vi "LogCycleHistory.vi"(8 "error in (no error)":errorcluster, 11 "Cycle History String Data In":string[](array[string])) -> (0 "error out":errorcluster)   [LabVIEW 2016]
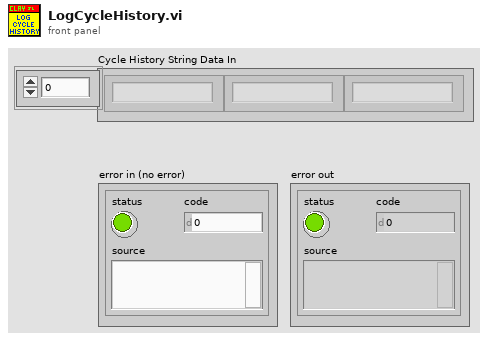
[diagram p1: front panel]
types:
  T1 = enum16{"open", "replace", "create", "open or create", "replace or create", "replace or create with confirmation"}
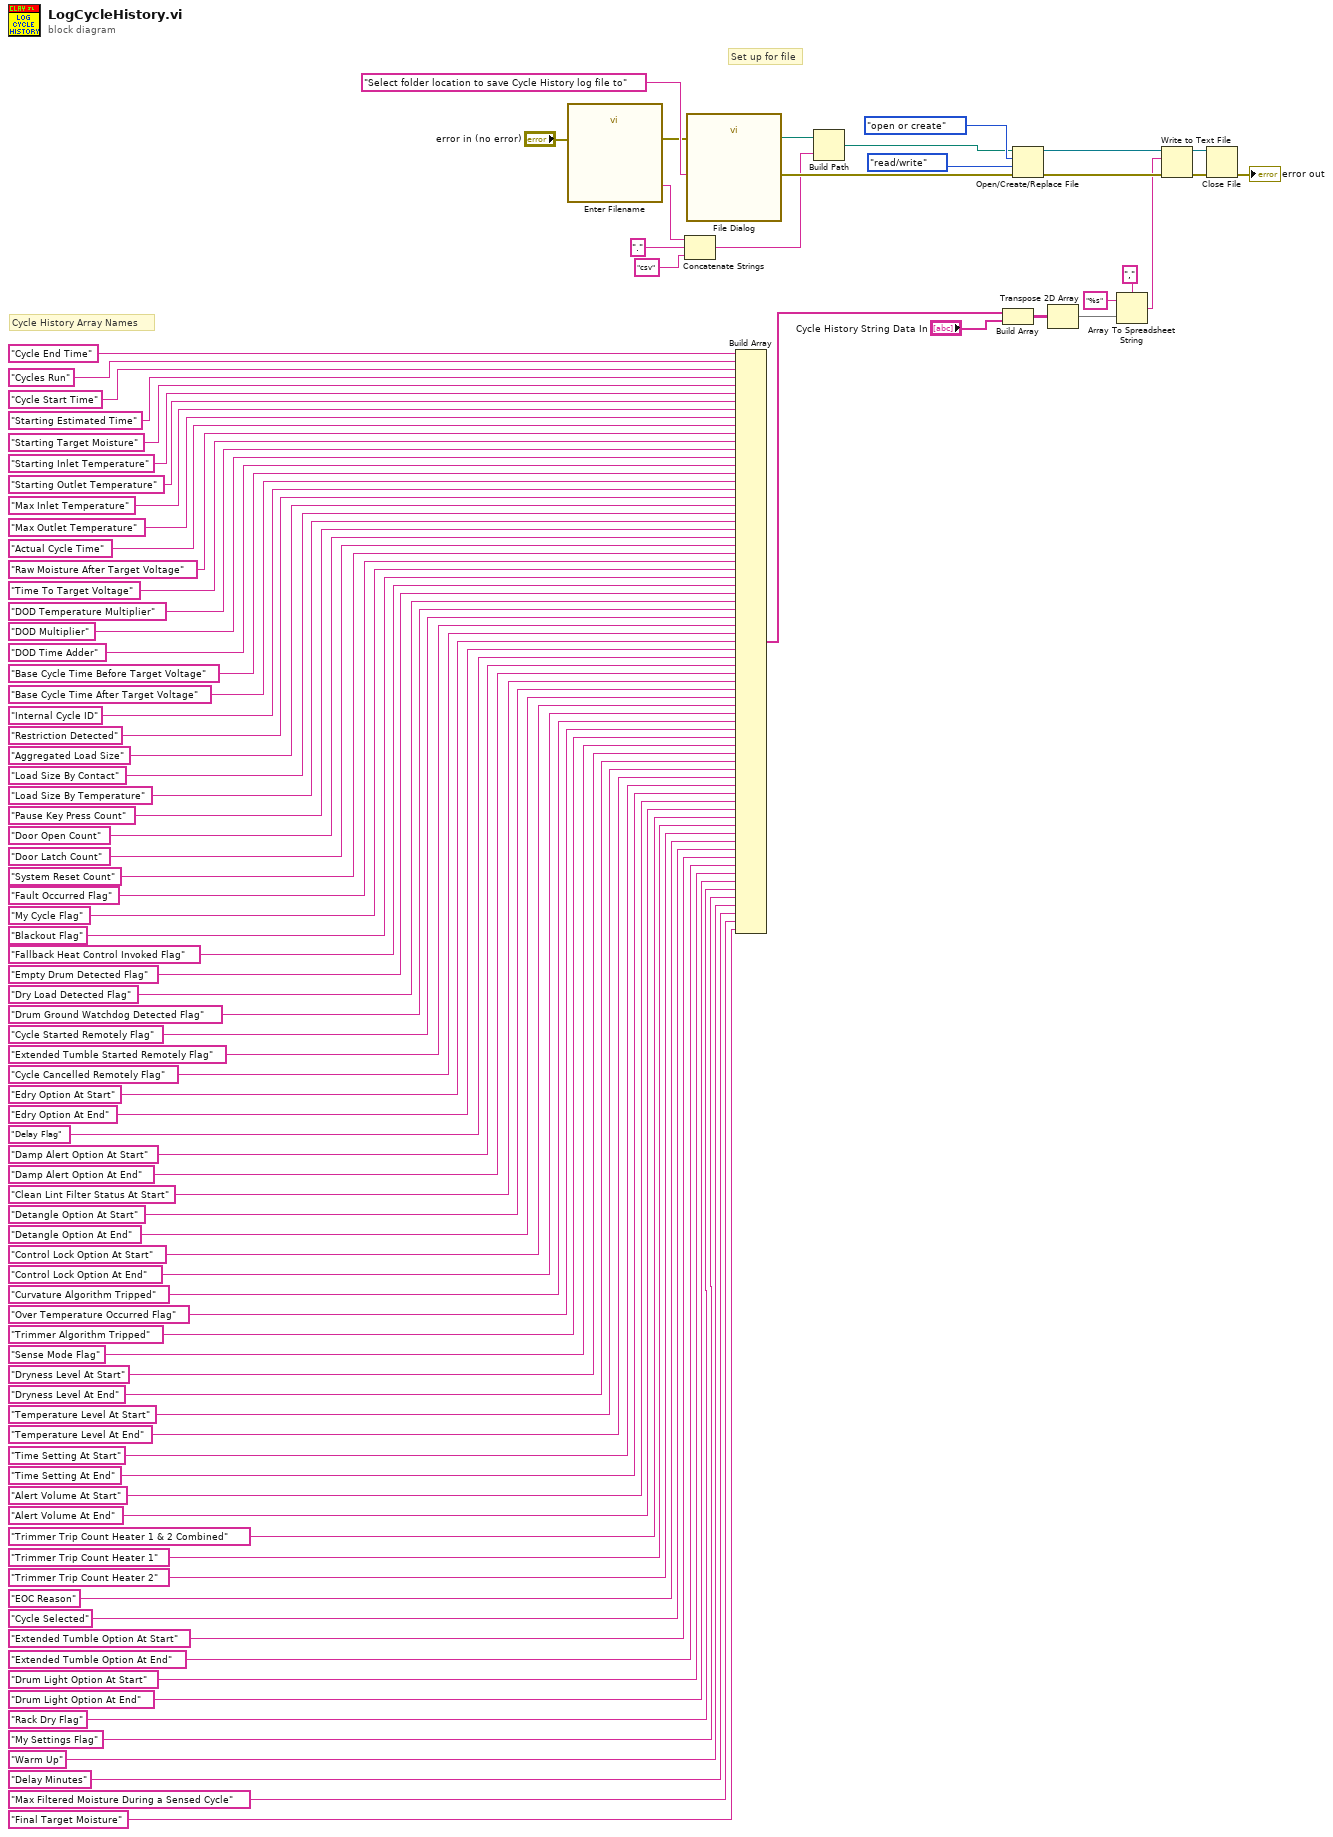
[diagram p0: block diagram]
diagram:
  # "Cycle History Array Names"
  # "Set up for file"
  n1 = call "Enter Filename"("error in (no error)"="error in (no error)") -> ("Filename"=w95:string, "error out"=w91:errorcluster)  [unwired: 16 in, 1 out]
  n2 = Concatenate Strings(w95, "." ("string"), "csv" ("string")) -> (w94:string)
  n3 = call "File Dialog"("prompt"="Select folder location to save Cycle History log file to", "error in"=w91) -> ("selected path"=w88:path, "error out"=w96:errorcluster)  [unwired: 10 in, 2 out]
  n4 = Build Array("Cycle End Time", "Cycles Run", "Cycle Start Time", "Starting Estimated Time", "Starting Target Moisture", "Starting Inlet Temperature", "Starting Outlet Temperature", "Max Inlet Temperature", "Max Outlet Temperature", "Actual Cycle Time", "Raw Moisture After Target Voltage", "Time To Target Voltage", "DOD Temperature Multiplier", "DOD Multiplier", "DOD Time Adder", "Base Cycle Time Before Target Voltage", "Base Cycle Time After Target Voltage", "Internal Cycle ID", "Restriction Detected", "Aggregated Load Size", "Load Size By Contact", "Load Size By Temperature", "Pause Key Press Count", "Door Open Count", "Door Latch Count", "System Reset Count", "Fault Occurred Flag", "My Cycle Flag", "Blackout Flag", "Fallback Heat Control Invoked Flag", "Empty Drum Detected Flag", "Dry Load Detected Flag", "Drum Ground Watchdog Detected Flag", "Cycle Started Remotely Flag", "Extended Tumble Started Remotely Flag", "Cycle Cancelled Remotely Flag", "Edry Option At Start", "Edry Option At End", "Delay Flag", "Damp Alert Option At Start", "Damp Alert Option At End", "Clean Lint Filter Status At Start", "Detangle Option At Start", "Detangle Option At End", "Control Lock Option At Start", "Control Lock Option At End", "Curvature Algorithm Tripped", "Over Temperature Occurred Flag", "Trimmer Algorithm Tripped", "Sense Mode Flag", "Dryness Level At Start", "Dryness Level At End", "Temperature Level At Start", "Temperature Level At End", "Time Setting At Start", "Time Setting At End", "Alert Volume At Start", "Alert Volume At End", "Trimmer Trip Count Heater 1 & 2 Combined", "Trimmer Trip Count Heater 1", "Trimmer Trip Count Heater 2", "EOC Reason", "Cycle Selected", "Extended Tumble Option At Start", "Extended Tumble Option At End", "Drum Light Option At Start", "Drum Light Option At End", "Rack Dry Flag", "My Settings Flag", "Warm Up", "Delay Minutes", "Max Filtered Moisture During a Sensed Cycle", "Final Target Moisture") -> (w4:string[])
  n5 = Build Path(base path=w88, name or relative path=w94) -> (appended path=w8:path)
  n6 = Build Array(w4, "Cycle History String Data In") -> (w6:string[][])
  n7 = Open/Create/Replace File(file path (use dialog)=w8, error in=w96, operation (0:open)=T1."open or create", access (0:read/write)=enum16{"read/write", "read-only", "write-only"}."read/write") -> (refnum out=w87:refnum<file>, error out=w86:errorcluster)  [unwired: 2 in, 1 out]
  n8 = Transpose 2D Array(2D array=w6) -> (transposed array=w5:string[][])
  n9 = Array To Spreadsheet String(delimiter (Tab)=",", array=w5, 3:"%s" ("format string")) -> (spreadsheet string=w82:string)
  n10 = Write to Text File(file (use dialog)=w87, text=w82, error in=w86) -> (refnum out=w85:refnum<file>, error out=w84:errorcluster)  [unwired: 1 in, 1 out]
  n11 = Close File(refnum=w85, error in=w84) -> (error out=→"error out":errorcluster)  [unwired: 1 out]
